vi "Rampdown Stop.vi"(8 "error in":errorcluster, 11 "Data Cluster":T1={"Chamber Address"={"Starting Address"=0, "Data Length"=0}, "Modbus RTU"={"unit ID"=1, "serial type"=enum."RTU", "baud rate"=9600, "parity (even)"=2, "flow control (none)"=0, "VISA resource name"=""}, "Temparature PASS?"=FALSE, "RMS Current PASS?"=FALSE, "Ping PASS?"=FALSE, "WaitMonitor_Class"=refnum, "Status Update"="", "Test Mode"=0, "Sequence Context"=refnum, "Running?"=FALSE, "RMS_FAIL_Count"=0, "Current Temperature"=0.0, "Target Temperature"=0.0, "RMS_Current"=[], "PowerStatus"={"Chamber IP Ping"=FALSE, "RAW_Power_Status"=FALSE, "PDU1_Status_Instrument_Rack"=FALSE, "PDU2_Status_PowerSupply_Rack_1"=FALSE, "PDU3_Status_PowerSupply_Rack_2"=FALSE}, "Monitor_Interval(S)"=0.0, "Current_Monitor_Interval(S)"=0.0, "RMS_Refresh?"=FALSE, "RTD Temperature(Deg C)"=0.0, "AbortTime(S)"=0.0, "HVPPS_Current"=[], "HVPPS Current PASS?"=FALSE} {"Modbus RTU"."parity (even)" items=["None", "Odd", "Even", "Mark", "Space"]; "Modbus RTU"."flow control (none)" items=["None", "XON/XOFF", "RTS/CTS", "XON/XOFF & RTS/CTS", "DTR/DSR", "XON/XOFF & DTR/DSR"]}) -> (0 "error out":errorcluster, 3 "Data Cluster out":T1={"Chamber Address"={"Starting Address"=0, "Data Length"=0}, "Modbus RTU"={"unit ID"=1, "serial type"=enum."RTU", "baud rate"=9600, "parity (even)"=2, "flow control (none)"=0, "VISA resource name"=""}, "Temparature PASS?"=FALSE, "RMS Current PASS?"=FALSE, "Ping PASS?"=FALSE, "WaitMonitor_Class"=refnum, "Status Update"="", "Test Mode"=0, "Sequence Context"=refnum, "Running?"=FALSE, "RMS_FAIL_Count"=0, "Current Temperature"=0.0, "Target Temperature"=0.0, "RMS_Current"=[], "PowerStatus"={"Chamber IP Ping"=FALSE, "RAW_Power_Status"=FALSE, "PDU1_Status_Instrument_Rack"=FALSE, "PDU2_Status_PowerSupply_Rack_1"=FALSE, "PDU3_Status_PowerSupply_Rack_2"=FALSE}, "Monitor_Interval(S)"=0.0, "Current_Monitor_Interval(S)"=0.0, "RMS_Refresh?"=FALSE, "RTD Temperature(Deg C)"=0.0, "AbortTime(S)"=0.0, "HVPPS_Current"=[], "HVPPS Current PASS?"=FALSE} {"Modbus RTU"."parity (even)" items=["None", "Odd", "Even", "Mark", "Space"]; "Modbus RTU"."flow control (none)" items=["None", "XON/XOFF", "RTS/CTS", "XON/XOFF & RTS/CTS", "DTR/DSR", "XON/XOFF & DTR/DSR"]})   [LabVIEW 2023, in "HardwareAbstractionLayer_LVOOP.lvlib" / "Wait Monitor.lvclass"]
uses:
  Wait Monitor.lvclass
  Control/Data Cluster.ctl
  <vilib>/addons/TestStand/_TSLegacy.llb/LabVIEW Test - Sequence Context.ctl
  Teststand Steptypes/PowerMonitor/Control/PowerData.ctl
  Teststand Steptypes/CAN/STP/Steptypes/Control/STP Data.ctl
  CAN/CAN Application Protocols/STP Protocol_class/Ctrls/STP CMD.ctl
  Teststand/Teststand.lvclass
  CAN/CAN Application Protocols/STP Protocol_class/STP Protocol.lvclass
  Teststand Steptypes/LTT_TeststandSteptypes.lvlib
panel:
  out "Positive Responce?":bool[](array[boolean])
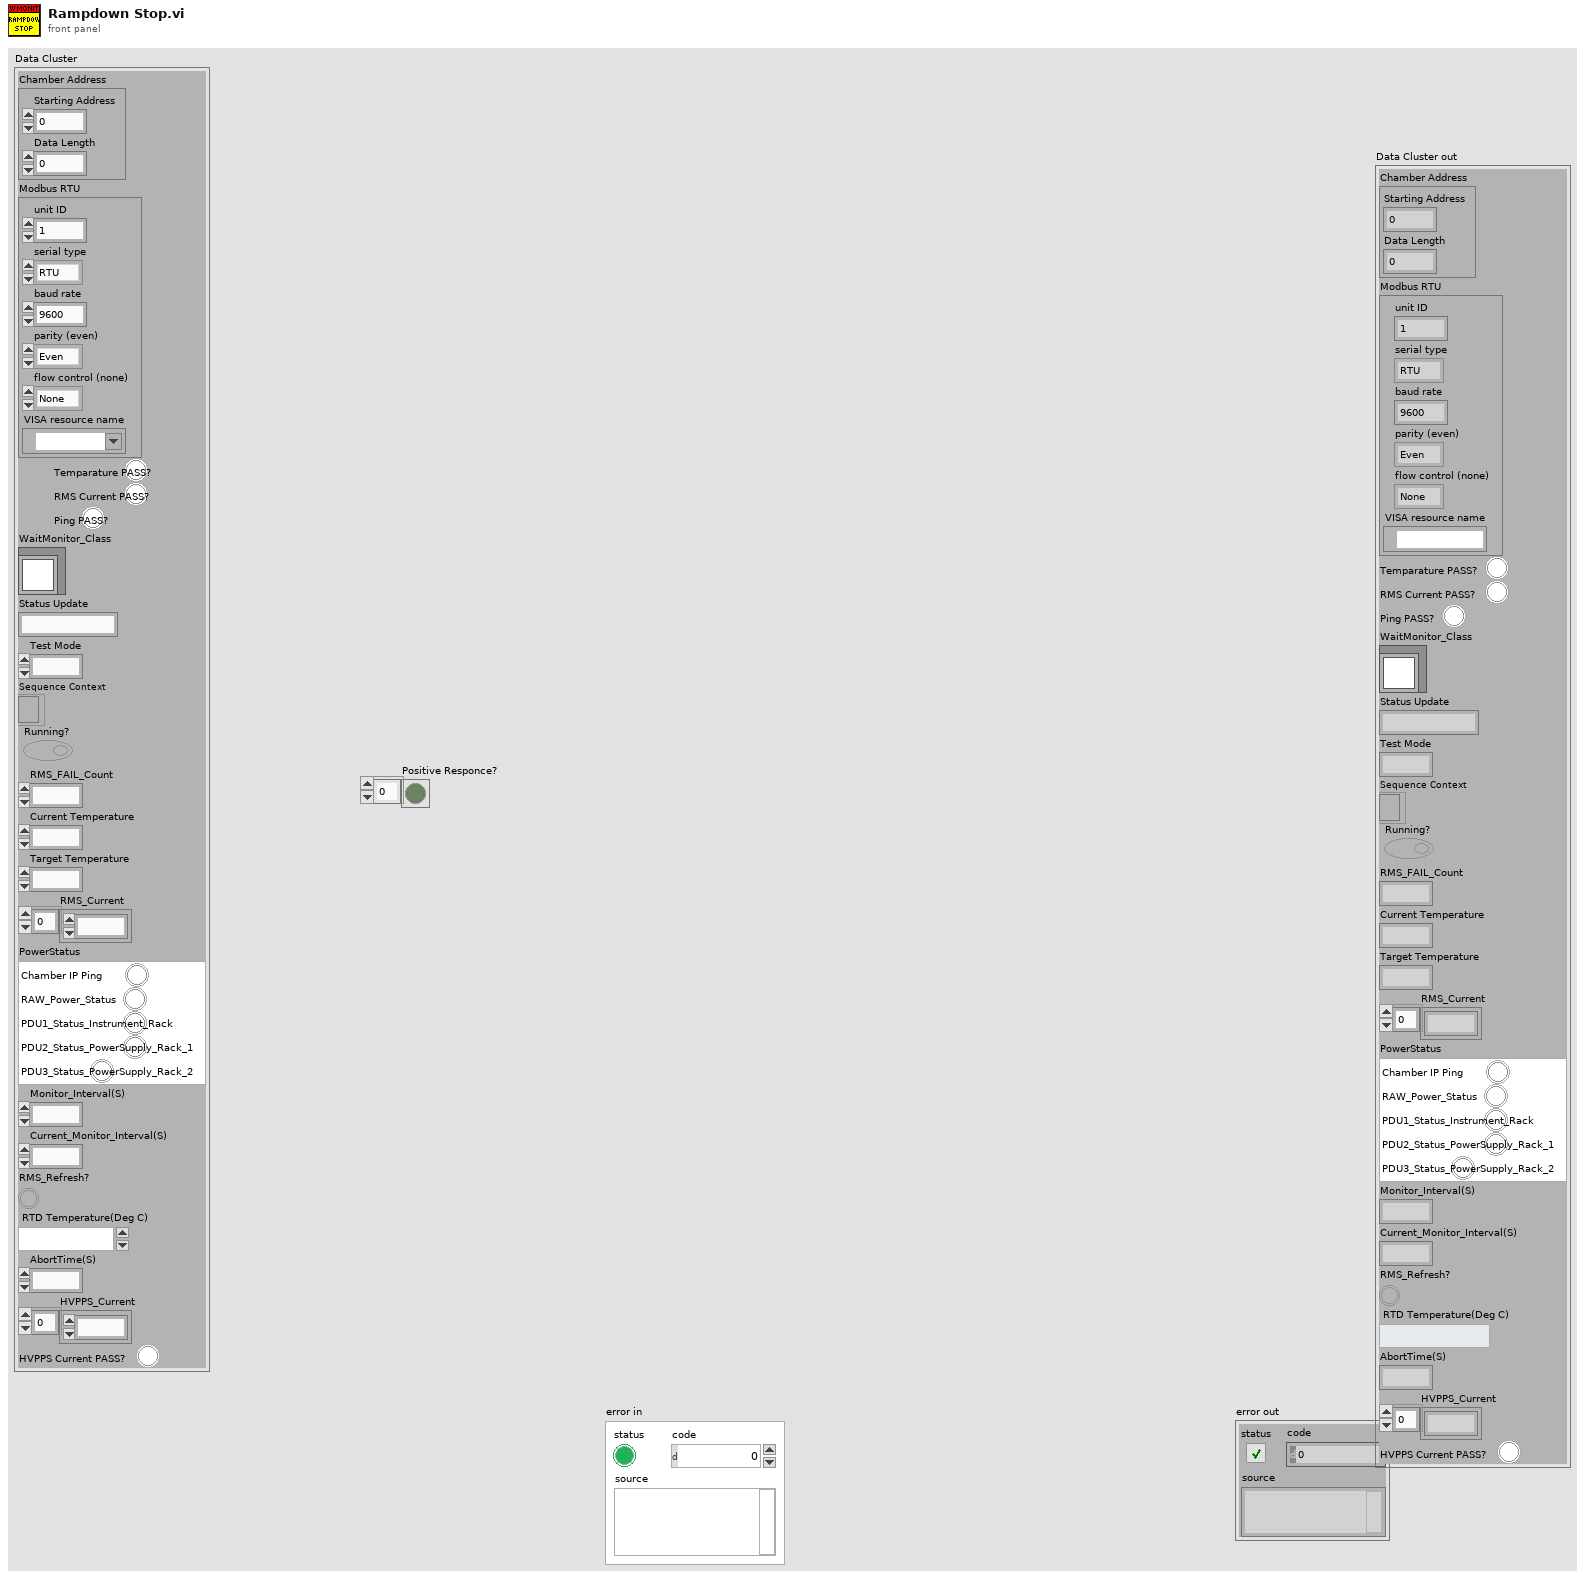
[diagram p1: front panel]
types:
  T1 = typedef "HardwareAbstractionLayer_LVOOP.lvlib/Wait Monitor.lvclass/Data Cluster.ctl" = cluster{"Chamber Address":cluster{"Starting Address":u16, "Data Length":u16}, "Modbus RTU":cluster{"unit ID":u8, "serial type":enum16{"RTU", "ASCII"}, "baud rate":u32, "parity (even)":u16, "flow control (none)":u16, "VISA resource name":refnum<visa-resource-name>}, "Temparature PASS?":bool, "RMS Current PASS?":bool, "Ping PASS?":bool, "WaitMonitor_Class":refnum<class "Wait Monitor.lvclass">, "Status Update":string, "Test Mode":u16, "Sequence Context":T2, "Running?":bool, "RMS_FAIL_Count":u16, "Current Temperature":dbl, "Target Temperature":dbl, "RMS_Current":dbl[], "PowerStatus":T3, "Monitor_Interval(S)":dbl, "Current_Monitor_Interval(S)":dbl, "RMS_Refresh?":bool, "RTD Temperature(Deg C)":dbl, "AbortTime(S)":dbl, "HVPPS_Current":dbl[], "HVPPS Current PASS?":bool}
  T2 = typedef "LabVIEW Test - Sequence Context.ctl" = refnum<k7>
  T3 = typedef "LTT_TeststandSteptypes.lvlib/PowerData.ctl" = cluster{"Chamber IP Ping":bool, "RAW_Power_Status":bool, "PDU1_Status_Instrument_Rack":bool, "PDU2_Status_PowerSupply_Rack_1":bool, "PDU3_Status_PowerSupply_Rack_2":bool}
  T4 = typedef "LTT_TeststandSteptypes.lvlib/STP Data.ctl" = cluster{"ECU CAN Port":string, "CMD":T5, "CAN Write Data":u8[], "Response Decoder":enum16{"String", "Number", "Boolean"}, "String":cluster{"Start Index":i32, "Length":i32}, "Number":cluster{"MSB Index":i32, "LSB Index":i32}, "Boolean":cluster{"Index":i32, "Bool":cluster{"7":bool, "6":bool, "5":bool, "4":bool, "3":bool, "2":bool, "1":bool, "0":bool, "7 Enabled":bool, "6 Enabled":bool, "5 Enabled":bool, "4 Enabled":bool, "3 Enabled":bool, "2 Enabled":bool, "1 Enabled":bool, "0 Enabled":bool}}}
  T5 = typedef "HardwareAbstractionLayer_LVOOP.lvlib/CAN Application Protocols Lib.lvlib/STP Protocol.lvclass/STP CMD.ctl" = u8
  T6 = typedef "HardwareAbstractionLayer_LVOOP.lvlib/Teststand.lvclass/Teststand Status Control.ctl" = cluster{"Terminating or Aborting":bool, "Stop":bool, "Socket Count":i16, "Selected Sockets":i16[]}
  T7 = typedef "LTT_TeststandSteptypes.lvlib/STP Out Data.ctl" = cluster{"String Data":string, "Numeric Data":dbl, "Boolean Data":bool, "RequestTimeout?":bool, "ResponseData":u8[], "PositiveResponse?":bool}
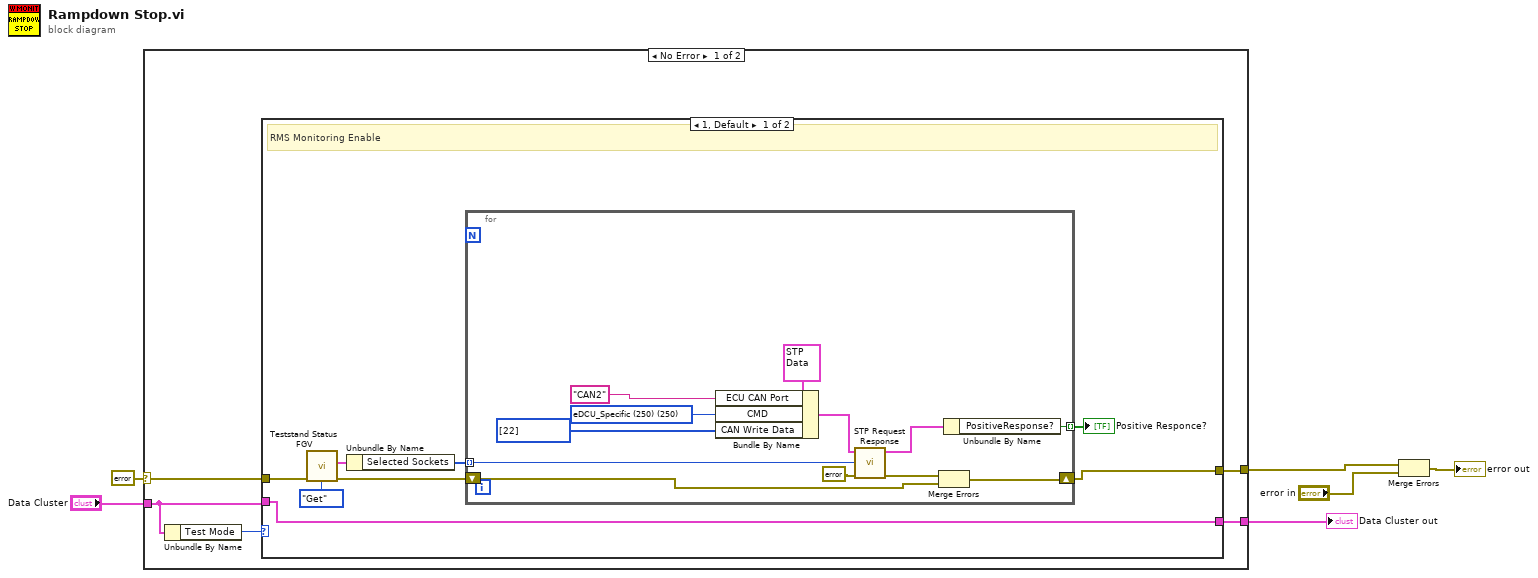
[diagram p0: block diagram]
diagram:
  n1 = case shown="No Error" errorcluster {"status"=FALSE, "code"=0, "source"=""} ("error IO") {
    selector: errorcluster {"status"=FALSE, "code"=0, "source"=""} ("error IO") -> [w7 w35]
    tunnel: [w11 w35] -> w6
    tunnel: "Data Cluster" -> [w9 w34]
    tunnel: [w10 w34] -> w4
    frame No Error {
      n2 = Unbundle By Name(w9) -> ("Test Mode"=w8:u16)
      n3 = case shown="1, Default" w8 {
        tunnel: w7 -> [w19 w33]
        tunnel: [w13 w33] -> w11
        tunnel: w9 -> [w18 w32]
        tunnel: [w18 w32] -> w10
        frame 1, Default {
          # "RMS Monitoring Enable"
          n4 = call "Teststand Status FGV.vi"("error in"=w19, "Option"=enum16{"Set", "Get"}."Get") -> ("error out"=w14:errorcluster, "Teststand Status Out"=w16:T6)  [unwired: 8 in]
          n5 = Unbundle By Name(w16) -> ("Selected Sockets"=w15:i16[])
          n6 = for {
            tunnel: w15 -> [w22] mode=indexing
            shift-right: [w23] -> w13
            shift-left: w14 -> [w31]
            tunnel: [w20] -> w12 mode=indexing
            w28 = T5 250 items=["TSW_VERSION(130)"=130, "WAIT_EVENT(132)"=132, "SEQUENCER(133)"=133, "TSW_RESET(150)"=150, "CONFIG_ECU(151)"=151, "TEST_CORE (152)"=152, "TEST_WATCHDOG (153)"=153, "TEST_MONITORING (154)"=154, "READ_MEMORY (162)"=162, "WRITE_ERASE_MEMORY (164)"=164, "COMM_EXTERNAL (190)"=190, "COMM_INTERNAL (195)"=195, "GET_ANALOG_INPUT (210)"=210, "GET_DIGITAL_INPUT (211)"=211, "GET_FREQUENCY_INPUT (212)"=212, "TEST_INPUT_STRUCTURE (214)"=214, "GENERATE_OUTPUT_SIGNAL (220)"=220, "GENERATE_SYNCHRONIZED_OUTPUT_SIGNALS (221)"=221, "eDCU_Specific (250)"=250] ("CMD")
            n7 = Bundle By Name(cluster=T4 {"ECU CAN Port"="CAN2", "CMD"=250, "CAN Write Data"=[34], "Response Decoder"=enum."String", "String"={"Start Index"=0, "Length"=-1}, "Number"={"MSB Index"=0, "LSB Index"=1}, "Boolean"={"Index"=0, "Bool"={"7"=FALSE, "6"=FALSE, "5"=FALSE, "4"=FALSE, "3"=FALSE, "2"=FALSE, "1"=FALSE, "0"=FALSE, "7 Enabled"=FALSE, "6 Enabled"=FALSE, "5 Enabled"=FALSE, "4 Enabled"=FALSE, "3 Enabled"=FALSE, "2 Enabled"=FALSE, "1 Enabled"=FALSE, "0 Enabled"=FALSE}}} ("STP Data in"), "ECU CAN Port"="CAN2", "CMD"=w28, "CAN Write Data"=u8[] [22]) -> (w24:T4)
            n8 = call "STP Request Response.vi"("error in"=errorcluster {"status"=FALSE, "code"=0, "source"=""}, "Socket No"=w22, "STP Data in"=w24) -> ("error out"=w30:errorcluster, "STP Data Out"=w21:T7)  [unwired: 5 in, 2 out]
            n9 = Merge Errors(w30, w31) -> (w23:errorcluster)
            n10 = Unbundle By Name(w21) -> ("PositiveResponse?"=w20:bool)
          }
          "Positive Responce?" <- w12
        }
        frame 0 {
        }
      }
    }
    frame Error {
    }
  }
  "Data Cluster out" <- w4
  n11 = Merge Errors(w6, "error in") -> (→"error out":errorcluster)
